vi "Close.vi"(8 "error in":errorcluster, 11 "Control Mode in":refnum<class "Control Mode.lvclass">) -> (0 "error out":errorcluster, 3 "Control Mode out":refnum<class "Control Mode.lvclass">)   [LabVIEW 2023, in "Control Mode.lvclass"]
uses:
  Control Mode.lvclass
  Control Mode.lvclass/Control Mode.ctl
  <vilib>/ADAS Replay HIL/AdasHilServices/AdasHilChannelServices.lvlib
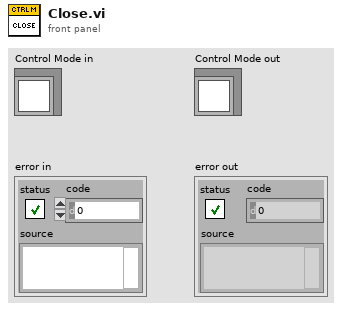
[diagram p1: front panel]
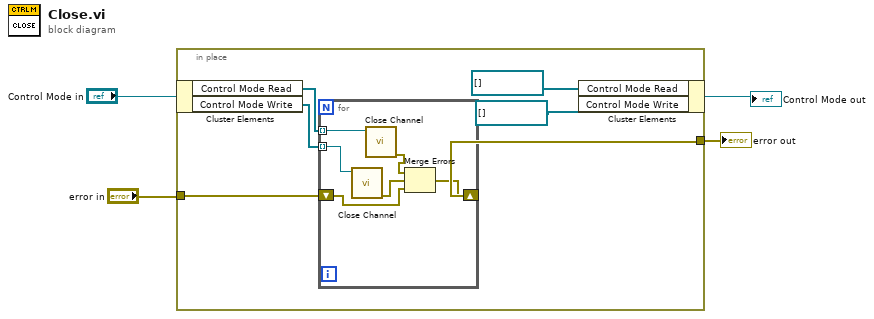
[diagram p0: block diagram]
diagram:
  n1 = in-place {
    in-place-border: "error in" -> [w10]
    in-place-border: [w9] -> w3
    n2 = in-place-cluster #1("Control Mode in") -> ("Control Mode Read"=w8:refnum<k21>[], "Control Mode Write"=w7:refnum<k21>[])
    n3 = for {
      tunnel: w8 -> [w16] mode=indexing
      tunnel: w7 -> [w15] mode=indexing
      shift-right: [w14] -> w9
      shift-left: w10 -> [w11]
      n4 = call <vilib>:"Close Channel.vi"("ADAS HIL Channel"=w15) -> ("error out"=w12:errorcluster)  [unwired: 10 in]
      n5 = call <vilib>:"Close Channel.vi"("ADAS HIL Channel"=w16) -> ("error out"=w13:errorcluster)  [unwired: 10 in]
      n6 = Merge Errors(w13, w12, w11) -> (w14:errorcluster)
    }
    n7 = in-place-cluster #1("Control Mode Read"=refnum<k21>[] [], "Control Mode Write"=refnum<k21>[] [] ("Control Mode Read")) -> (→"Control Mode out":refnum<class "Control Mode.lvclass">)
  }
  "error out" <- w3
